vi "Continuous Sound Input.vi"() -> ()   [LabVIEW 2017]
doc: "本VI说明了从指定设备连续采集声音采样的方式。需要使用连接至声卡的麦克风。可指定需采集的采样数、采样率、通道数和每采样比特率。本VI也将在采样时绘制原始数据。"
uses:
  <vilib>/sound2/lvsound2.llb/Sampling Mode.ctl
  <vilib>/sound2/lvsound2.llb/Sound Data Format.ctl
  <vilib>/sound2/lvsound2.llb/Sound Input Read (DBL).vi
panel:
  in  "设备ID":u32 format="%.0x"
  in  "每通道采样数":i32=5000
  out "原始数据":waveform(dbl)[](graph)
  in  "停止":bool
  # "概述：演示通过声音输入函数使用连接至声卡的麦克风连续采集声音采样。\n要求：麦克风\n操作步骤：\n1.指定设备ID和每通道采样数的值。\n2.运行VI。\n3.VI将连续采样并将原始数据绘制到图形。\n4.单击停止按钮停止VI。"
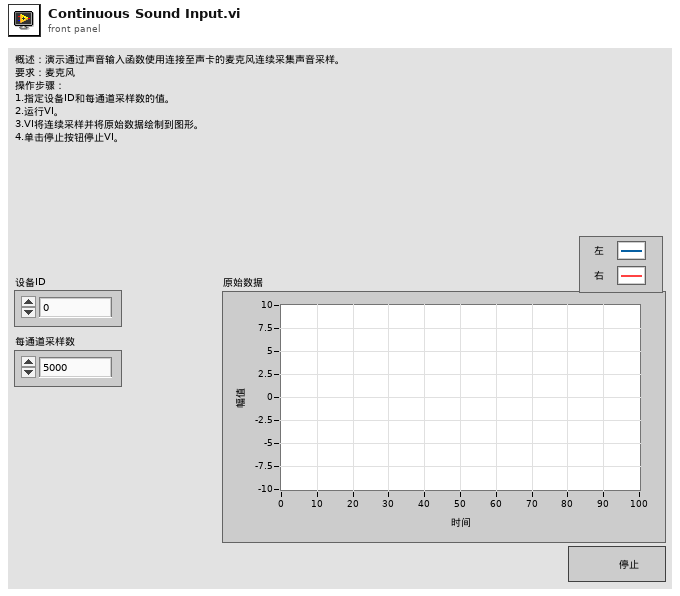
[diagram p1: front panel]
types:
  T1 = typedef "Sound Data Format.ctl" = cluster{"sample rate (S/s)":dbl, "number of channels":i32, "bits per sample":i32}
  T2 = typedef "Sampling Mode.ctl" = i32
  T3 = typedef "Sound Input Task ID.ctl" = u32
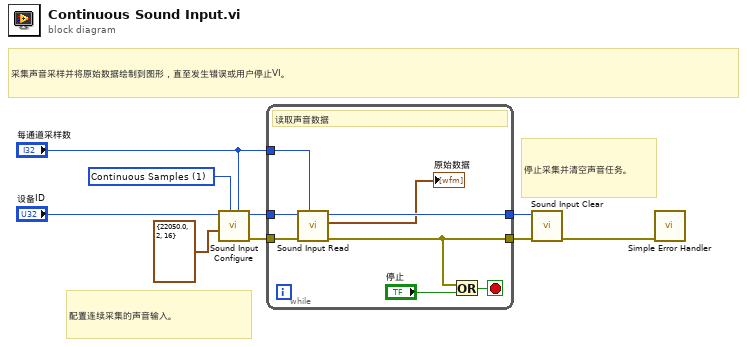
[diagram p0: block diagram]
diagram:
  w4 = T2 1 items=["Finite Samples", "Continuous Samples"] ("sample mode")
  # "采集声音采样并将原始数据绘制到图形，直至发生错误或用户停止VI。"
  # "停止采集并清空声音任务。"
  # "配置连续采集的声音输入。"
  n1 = call <vilib>:"Sound Input Configure.vi"("number of samples/ch"="每通道采样数", "sample mode"=w4, "sound format"=T1 {"sample rate (S/s)"=22050.0, "number of channels"=2, "bits per sample"=16} ("Sound Format"), "device ID"="设备ID") -> ("error out"=w9:errorcluster, "task ID"=w7:T3)  [unwired: 6 in]
  n2 = while {
    tunnel: w7 -> [w16]
    tunnel: [w15] -> w6
    tunnel: "每通道采样数" -> [w14]
    tunnel: w9 -> [w17]
    tunnel: [w10] -> w5
    stop <- w12 stop-if-true
    # "读取声音数据"
    n3 = call-poly <vilib>:"Sound Input Read.vi"("number of samples/ch"=w14, "error in (no error)"=w17, "task ID"=w16) -> ("error out"=w10:errorcluster, "data"=→"原始数据":waveform(dbl)[], "task ID out"=w15:T3)  [unwired: 6 in]
    n4 = Or(x=w10, y="停止") -> (x .or. y?=w12:bool)
  }
  n5 = call <vilib>:"Sound Input Clear.vi"("error in (no error)"=w5, "task ID"=w6) -> ("error out"=w2:errorcluster)  [unwired: 9 in]
  n6 = call <vilib>:"Simple Error Handler.vi"("error in (no error)"=w2) -> ()  [unwired: 4 in, 5 out]
